vi "Close.vi"(8 "error in (no error)":errorcluster, 11 "Yokogawa WT1600 in":refnum<class "Yokogawa WT1600.lvclass">) -> (0 "error out":errorcluster, 2 "VISA resource name":refnum<visa-resource-name>, 3 "Yokogawa WT1600 out":refnum<class "Yokogawa WT1600.lvclass">)   [LabVIEW 2013, in "Universal Power Meter.lvlib" / "Yokogawa WT1600.lvlib" / "Yokogawa WT1600.lvclass"]
uses:
  Yokogawa WT1600.lvclass
  Universal Power Meter class/Universal Power Meter.lvclass
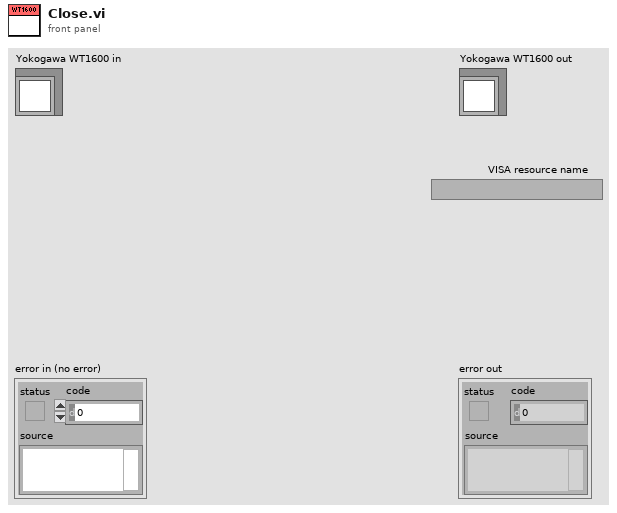
[diagram p1: front panel]
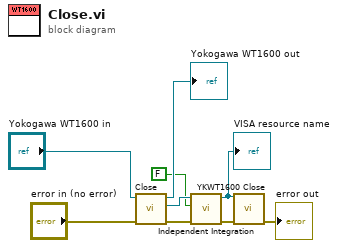
[diagram p0: block diagram]
diagram:
  n1 = call-parent "Close.vi"("error in (no error)"="error in (no error)", "Universal Power Meter in"="Yokogawa WT1600 in") -> ("error out"=w4:errorcluster, "VISA resource name"=w5:refnum<visa-resource-name>, "Universal Power Meter out"=→"Yokogawa WT1600 out":refnum<class "Yokogawa WT1600.lvclass">)  [unwired: 7 in]
  n2 = call "Independent Integration.vi"("error in"=w4, "ON/OFF"=FALSE, "VISA resource name"=w5) -> ("error out"=w3:errorcluster, "VISA resource name out"=w2:refnum<visa-resource-name>)  [unwired: 7 in]
  "VISA resource name" <- w2
  n3 = call <instrlib>:"YKWT1600 Close.vi"("VISA session"=w2, "error in (no error)"=w3) -> ("error out"=→"error out":errorcluster)  [unwired: 13 in]
